vi "Test Create.vi"() -> ()   [LabVIEW 2014, in "Arduino SoftwareSerial Wrapper.lvlib"]
uses:
  Arduino SoftwareSerial Wrapper.lvlib
panel:
  out "Error Out":errorcluster
  in  "Error In":errorcluster
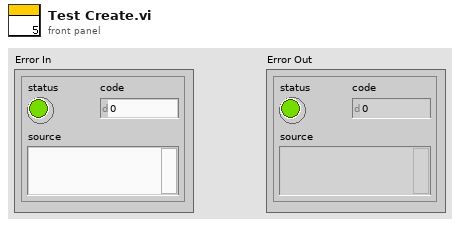
[diagram p1: front panel]
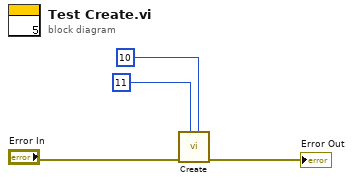
[diagram p0: block diagram]
diagram:
  n1 = call "Create.vi"("arduino RX pin"=u8 10 ("RX pin"), "arduino TX pin"=u8 11 ("RX pin"), "Error In"="Error In") -> ("Error Out"=→"Error Out":errorcluster)  [unwired: 8 in]
